vi "Connect_ID_Search.vi"(8 "error in":errorcluster, 11 "channel":T1) -> (0 "error out":errorcluster, 3 "Arduino Ref":refnum<visa-resource-name>)   [LabVIEW 2019]
uses:
  <extravilib>/ChannelInstances/Tag-bool/))Channel.ctl
  <vilib>/Instr/_visa.llb/VISA Find Search Mode.ctl
  99c092ff-e2f7-4cbe-ac4a-4332005b7ad8.vi
  de12ef85-3502-42e1-b281-974d967aa2b5.vi
  <extravilib>/ChannelInstances/Tag-bool/Read With Abort.vi
  <extravilib>/ChannelInstances/Tag-bool/EndpointRead.vi
  <vilib>/Instr/_visa.llb/VISA Configure Serial Port (Instr).vi
  <extravilib>/ChannelInstances/Tag-bool.lvlib
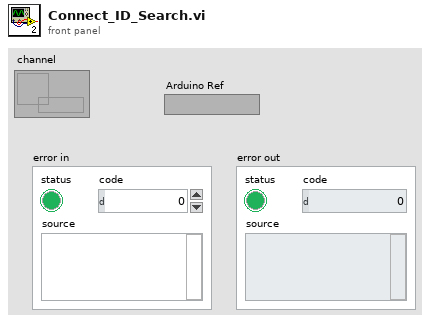
[diagram p1: front panel]
types:
  T1 = typedef "Tag-bool.lvlib/))Channel.ctl" = refnum<queue>
  T2 = typedef "VISA Find Search Mode.ctl" = u32
  T3 = cluster{"value out":refnum<visa-resource-name>, "error out":errorcluster}
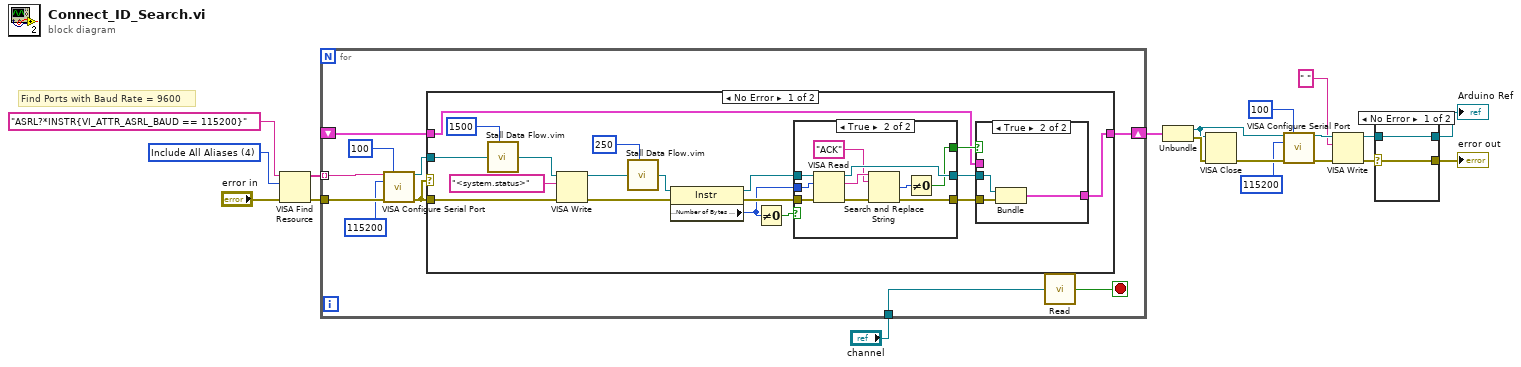
[diagram p0: block diagram]
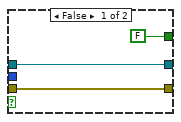
[diagram p3: hidden frame]
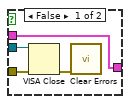
[diagram p4: hidden frame]
diagram:
  w9 = T2 4 items=["Canonical Names Only"=0, "Aliases Only"=2, "Include Matching Aliases"=3, "Include All Aliases"=4] ("Search Mode")
  # "Find Ports with Baud Rate = 9600"
  n1 = VISA Find Resource(8:"error in", 10:w9, 11:"ASRL?*INSTR{VI_ATTR_ASRL_BAUD == 115200}" ("expression (\"?*\")")) -> (0:w18:errorcluster, 3:w3:string[])  [unwired: 1 out]
  n2 = for {
    tunnel: w3 -> [w26] mode=indexing
    shift-right: [w29] -> w19
    shift-left: _ -> [w27]
    tunnel: w18 -> [w25]
    tunnel: "channel" -> [w21]
    stop <- w22 stop-if-true
    n3 = call-poly "VISA Configure Serial Port"("VISA resource name"=w26, "timeout (10sec)"=u32 100 ("VISA Open timeout (0)"), "baud rate (9600)"=u32 115200, "error in (no error)"=w25) -> ("VISA resource name out"=w23:refnum<visa-resource-name>, "error out"=w24:errorcluster)  [unwired: 10 in]
    n4 = case shown="No Error" w24 {
      tunnel: [w47 w68] -> w29
      tunnel: w24 -> [w46 _]
      tunnel: w27 -> [w36 w68]
      tunnel: w23 -> [w32 _]
      frame No Error {
        n5 = call "Stall Data Flow.vim"("value in"=w32, "milliseconds to wait"=u32 1500) -> ("value out"=w31:refnum<visa-resource-name>)  [unwired: 1 out]
        n6 = VISA Write(VISA resource name=w31, write buffer="<system.status>", error in (no error)=w46) -> (VISA resource name out=w45:refnum<visa-resource-name>, error out=w44:errorcluster)  [unwired: 1 out]
        n7 = call "Stall Data Flow.vim"("value in"=w45, "milliseconds to wait"=u32 250) -> ("value out"=w35:refnum<visa-resource-name>)  [unwired: 1 out]
        n8 = property class="Instr"(reference=w35, error in=w44) -> (reference out=w42:refnum<visa-resource-name>, error out=w41:errorcluster, "Serial Settings:Number of Bytes at Serial Port"=w37:u32)
        n9 = Not Equal To 0?(x=w37) -> (x != 0?=w43:bool)
        n10 = case shown="True" w43 {
          tunnel: [w50 w60] -> w39
          tunnel: w42 -> [w50 w59]
          tunnel: w37 -> [_ w58]
          tunnel: [FALSE w54] -> w40
          tunnel: w41 -> [w48 w53]
          tunnel: [w48 w51] -> w38
          frame False {
          }
          frame True {
            n11 = VISA Read(VISA resource name=w59, byte count=w58, error in (no error)=w53) -> (VISA resource name out=w60:refnum<visa-resource-name>, read buffer=w56:string, error out=w52:errorcluster)  [unwired: 1 out]
            n12 = Search and Replace String(input string=w56, search string="ACK", error in=w52) -> (number of replacements=w57:i32, error out=w51:errorcluster)  [unwired: 5 in, 2 out]
            n13 = Not Equal To 0?(x=w57) -> (x != 0?=w54:bool)
          }
        }
        n14 = case shown="True" w40 {
          tunnel: [w64 w67] -> w47
          tunnel: w39 -> [w63 w66]
          tunnel: w38 -> [w62 w65]
          tunnel: w36 -> [w64 _]
          frame False {
            n15 = VISA Close(VISA resource name=w63, error in (no error)=w62) -> (error out=w61:errorcluster)
            n16 = call <vilib>:"Clear Errors.vi"("error in (no error)"=w61) -> ()  [unwired: 5 in, 2 out]
          }
          frame True {
            n17 = Bundle("value out"=w66, "error out"=w65) -> (w67:T3)  [unwired: 1 in]
          }
        }
      }
      frame Error {
      }
    }
    n18 = call <extravilib>:"Read.vi"("channel"=w21) -> ("element"=w22:bool)  [unwired: 1 in, 1 out]
  }
  n19 = Unbundle(w19) -> ("value out"=w10:refnum<visa-resource-name>, "error out"=w15:errorcluster)
  n20 = VISA Close(VISA resource name=w10, error in (no error)=w15) -> (error out=w14:errorcluster)
  n21 = call-poly "VISA Configure Serial Port"("VISA resource name"=w10, "timeout (10sec)"=u32 100, "baud rate (9600)"=u32 115200, "error in (no error)"=w14) -> ("VISA resource name out"=w13:refnum<visa-resource-name>, "error out"=w12:errorcluster)  [unwired: 10 in]
  n22 = VISA Write(VISA resource name=w13, write buffer=" ", error in (no error)=w12) -> (VISA resource name out=w8:refnum<visa-resource-name>, error out=w7:errorcluster)  [unwired: 1 out]
  n23 = case shown="No Error" w7 {
    selector: w7 -> [w69 w71]
    tunnel: w8 -> [w70 _]
    tunnel: [w70 _] -> w5
    tunnel: [w69 w71] -> w6
    frame No Error {
    }
    frame Error {
    }
  }
  "Arduino Ref" <- w5
  "error out" <- w6
